vi "ToRepo.vi"(8 "error in":errorcluster, 9 "to repo cluster":T1, 10 "repository in":refnum<class "NISE_CEF_Repository.lvclass">, 11 "SequenceNode in":refnum<class "CleanupCategoryNode.lvclass">) -> (0 "error out":errorcluster, 2 "repository out":refnum<class "NISE_CEF_Repository.lvclass">, 3 "SequenceNode out":refnum<class "CleanupCategoryNode.lvclass">)   [LabVIEW 2015, in "CleanupCategoryNode.lvclass"]
doc: "Copyright 2017 National Instruments Corporation\n\nLicensed under the Apache License, Version 2.0 (the \"License\"); you may not use this file except in compliance with the License. You may obtain a copy of the License at http://www.apache.org/licenses/LICENSE-2.0\nUnless required by applicable law or agreed to in writing, software distributed under the License is distributed on an \"AS IS\" BASIS, WITHOUT WARRANTIES OR CONDITIONS OF ANY KIND, either express or implied. See the License for the specific language governing permissions and limitations under the License."
uses:
  CleanupCategoryNode.lvclass
  <vilib>/NI/Configuration Framework/Repository/NISE_CEF_Repository.lvclass
  <vilib>/NI/Configuration Framework/Node/ToRepoCluster.ctl
  SequenceRepo/SequenceRepo.lvclass
  Prototype/classes/Step/Config/Step Config.lvclass
  Prototype/classes/Sequence/Config/Sequence Config.lvclass
  <vilib>/NI/Configuration Framework/Node/NISE_CEF_Node.lvclass
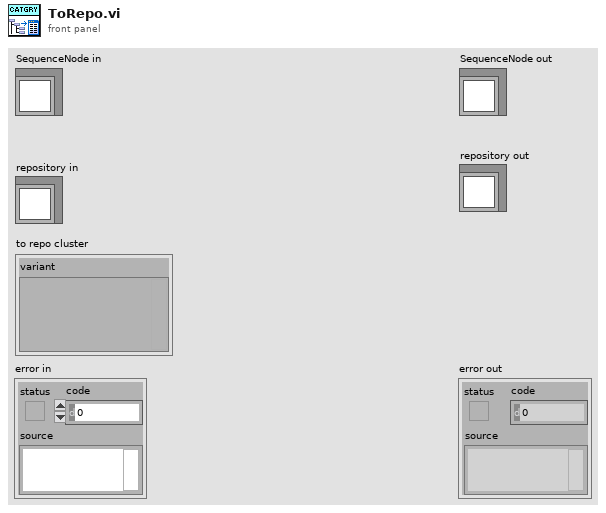
[diagram p1: front panel]
types:
  T1 = typedef "NISE_CEF_Node.lvclass/ToRepoCluster.ctl" = cluster{"variant":variant}
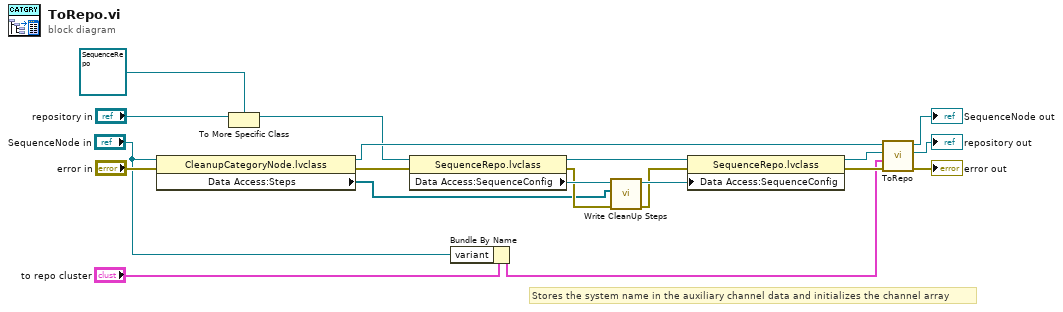
[diagram p0: block diagram]
diagram:
  # "Stores the system name in the auxiliary channel data and initializes the channel array"
  n1 = property class="CleanupCategoryNode.lvclass"(reference="SequenceNode in", error in="error in") -> (reference out=w14:refnum<class "CleanupCategoryNode.lvclass">, error out=w12:errorcluster, "Data Access:Steps"=w3:refnum<class "Step Config.lvclass">[])
  n2 = To More Specific Class(target class=refnum<class "SequenceRepo.lvclass"> refnum ("cRIO repo.lvclass"), reference="repository in") -> (specific class reference=w9:refnum<class "SequenceRepo.lvclass">)  [unwired: 1 in, 1 out]
  n3 = property class="SequenceRepo.lvclass"(reference=w9, error in=w12) -> (reference out=w8:refnum<class "SequenceRepo.lvclass">, error out=w5:errorcluster, "Data Access:SequenceConfig"=w7:refnum<class "Sequence Config.lvclass">)
  n4 = Bundle By Name(cluster="to repo cluster", "variant"="SequenceNode in") -> (w2:T1)
  n5 = call-dynamic "Write CleanUp Steps .vi"("error in (no error)"=w5, "CleanUp Steps"=w3, "Sequence Config in"=w7) -> ("error out"=w4:errorcluster, "Sequence Config out"=w6:refnum<class "Sequence Config.lvclass">)  [unwired: 7 in]
  n6 = property class="SequenceRepo.lvclass"(reference=w8, error in=w4, "Data Access:SequenceConfig"=w6) -> (reference out=w17:refnum<class "SequenceRepo.lvclass">, error out=w11:errorcluster)
  n7 = call-parent "ToRepo.vi"("error in"=w11, "to repo cluster"=w2, "repository in"=w17, "node in"=w14) -> ("error out"=→"error out":errorcluster, "repository out"=→"repository out":refnum<class "NISE_CEF_Repository.lvclass">, "node out"=→"SequenceNode out":refnum<class "CleanupCategoryNode.lvclass">)  [unwired: 5 in]
